vi "Read paramHigh.vi"(8 "error in (no error)":errorcluster, 11 "ApplicationEvent in":refnum<class "ApplicationEvent.lvclass">) -> (0 "error out":errorcluster, 2 "paramHigh":u16, 3 "ApplicationEvent out":refnum<class "ApplicationEvent.lvclass">)   [LabVIEW 2013, in "MaterialCharacterization.lvlib" / "ApplicationEvent.lvclass"]
uses:
  ApplicationEvent.lvclass
  ApplicationEvent.lvclass/ApplicationEvent.ctl
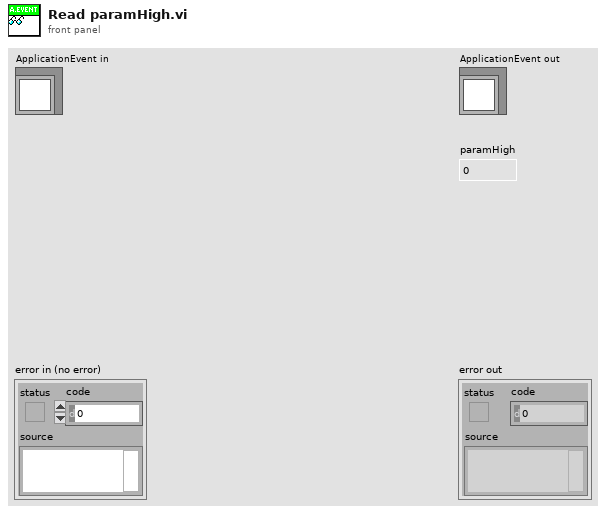
[diagram p1: front panel]
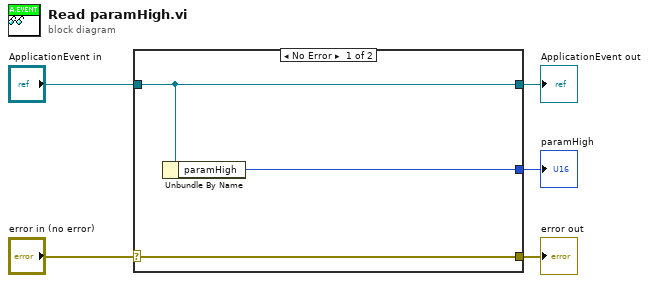
[diagram p0: block diagram]
diagram:
  n1 = case shown="No Error" "error in (no error)" {
    selector: "error in (no error)" -> [w8 w9]
    tunnel: [w8 w9] -> w4
    tunnel: [w7 w10] -> w2
    tunnel: "ApplicationEvent in" -> [w7 w10]
    tunnel: [w6 _] -> w1
    frame No Error {
      n2 = Unbundle By Name(w7) -> ("paramHigh"=w6:u16)
    }
    frame Error {
    }
  }
  "error out" <- w4
  "ApplicationEvent out" <- w2
  "paramHigh" <- w1
